vi "Stop TCS.vi"(8 "error in (no error)":errorcluster, 11 "SPARC4_GEI in":refnum<class "S4GEI.lvclass">) -> (0 "error out":errorcluster, 3 "SPARC4_GEI out":refnum<class "S4GEI.lvclass">)   [LabVIEW 2018, in "S4GEI.lvclass"]
uses:
  S4GEI.lvclass
  TCS/TCS.lvclass
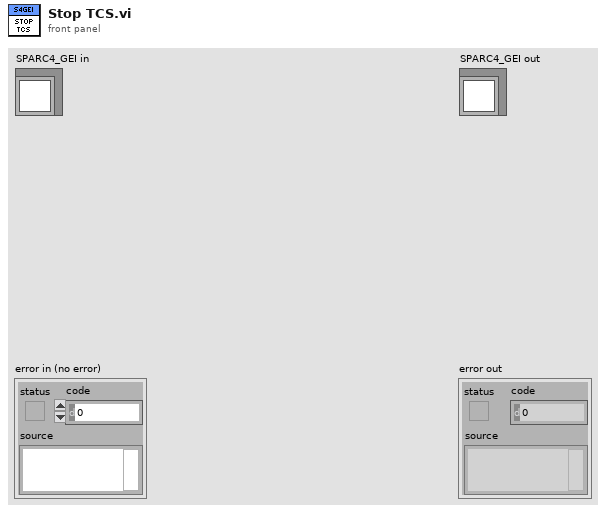
[diagram p1: front panel]
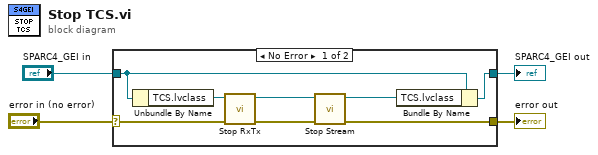
[diagram p0: block diagram]
diagram:
  n1 = case shown="No Error" "error in (no error)" {
    selector: "error in (no error)" -> [w8 w14]
    tunnel: [w5 w14] -> w3
    tunnel: [w11 w13] -> w1
    tunnel: "SPARC4_GEI in" -> [w12 w13]
    frame No Error {
      n2 = Unbundle By Name(w12) -> ("TCS.lvclass"=w7:refnum<class "TCS.lvclass">)
      n3 = call "Stop RxTx.vi"("error in (no error)"=w8, "TCS in"=w7) -> ("error out"=w10:errorcluster, "TCS out"=w9:refnum<class "TCS.lvclass">)  [unwired: 8 in]
      n4 = call "Stop Stream.vi"("error in (no error)"=w10, "TCS in"=w9) -> ("error out"=w5:errorcluster, "TCS out"=w6:refnum<class "TCS.lvclass">)  [unwired: 8 in]
      n5 = Bundle By Name(cluster=w12, "TCS.lvclass"=w6) -> (w11:refnum<class "S4GEI.lvclass">)
    }
    frame Error {
    }
  }
  "error out" <- w3
  "SPARC4_GEI out" <- w1
